vi "BiasPreamp.vi"(0 "VISA resource name":refnum<visa-resource-name>="COM8", 1 "CHANGE SENS?":bool=TRUE, 2 "Sensitivity":T1(ring)=enum."100nA/V", 3 "Bias on":bool=TRUE, 4 "Bias Voltage (mv)":i32=-25) -> ()   [LabVIEW 2013]
uses:
  <vilib>/Instr/_visa.llb/VISA Configure Serial Port (Instr).vi
panel:
  in  "flow control":u16(ring) items=["None"=0, "XON/XOFF"=1, "RTS/CTS"=2, "DTR/DSR"=4]
  in  "stop bits":u16(ring)=10 items=["1.0"=10, "1.5"=15, "2.0"=20]
  in  "parity":u16(ring) items=["None", "Odd", "Even", "Mark", "Space"]
  in  "data bits":u16=8 min=5 max=8 step=1
  in  "baud rate":u32=9600
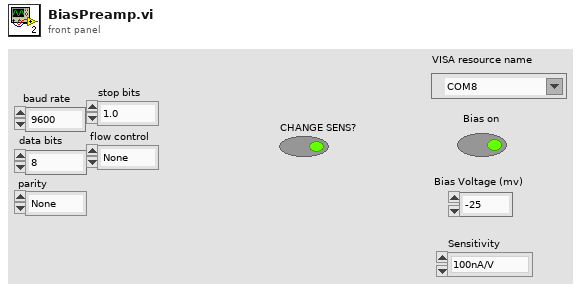
[diagram p1: front panel]
types:
  T1 = enum16{"1pA/V", "2pA/V", "5pA/V", "10pA/V", "20pA/V", "50pA/V", "100pA/V", "200pA/V", "500pA/V", "1nA/V", "2nA/V", "5nA/V", "10nA/V", "20nA/V", "50nA/V", "100nA/V", "200nA/V", "500nA/V", "1uA/V", "2uA/V", "5uA/V", "10uA/V", "20uA/V", "50uA/V", "100uA/V", "200uA/V", "500uA/V", "1mA/V"}
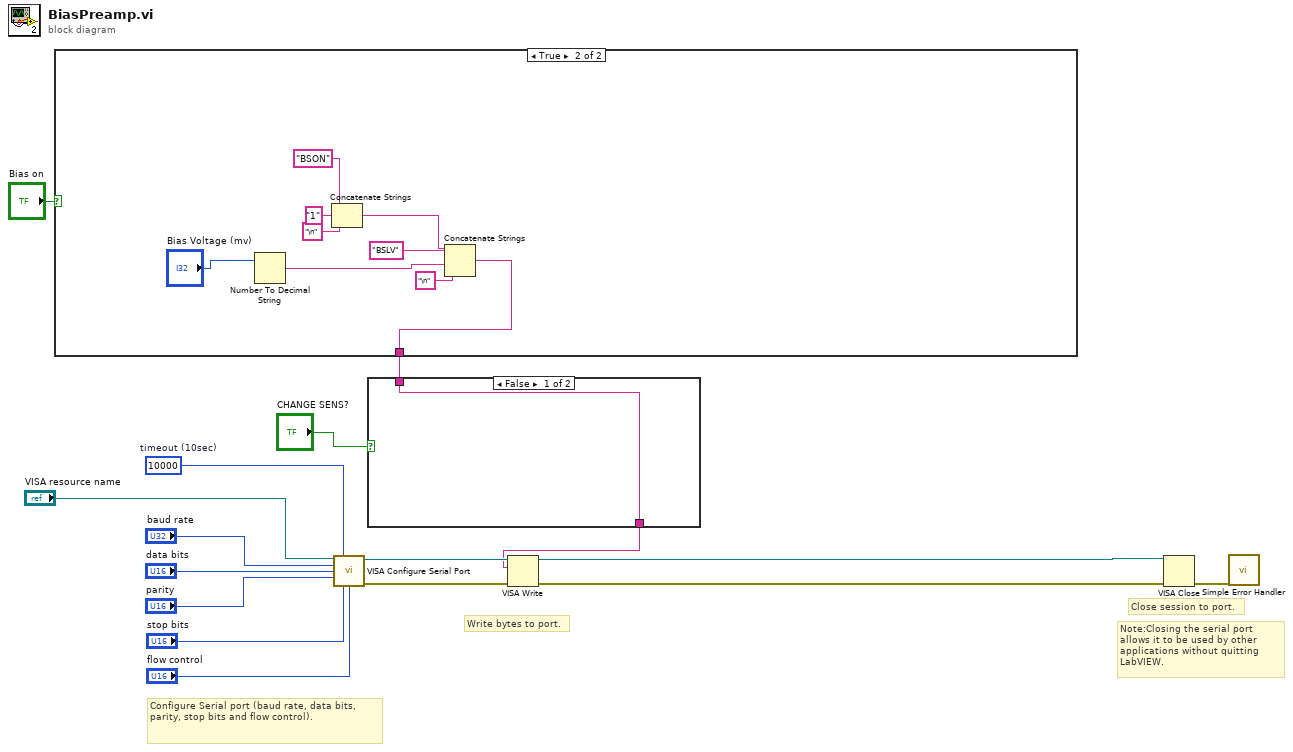
[diagram p0: block diagram]
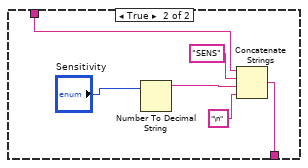
[diagram p2: hidden frame]
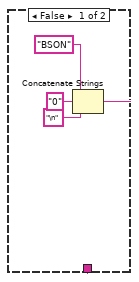
[diagram p3: hidden frame]
diagram:
  w10 = u32 10000  # timeout (10sec)
  # "Write bytes to port."
  # "Note:Closing the serial port allows it to be used by other applications without quitting LabVIEW."
  # "Configure Serial port (baud rate, data bits, parity, stop bits and flow control)."
  # "Close session to port."
  n1 = case shown="True" "Bias on" {
    tunnel: [w17 w22] -> w3
    frame False {
      n2 = Concatenate Strings("BSON", "0" ("string"), "\n" ("string")) -> (w17:string)
    }
    frame True {
      n3 = Number To Decimal String(number="Bias Voltage (mv)") -> (decimal integer string=w23:string)  [unwired: 1 in]
      n4 = Concatenate Strings("BSON", "1" ("string"), "\n" ("string")) -> (w21:string)
      n5 = Concatenate Strings(w21, "BSLV", w23, "\n" ("string")) -> (w22:string)
    }
  }
  n6 = call-poly "VISA Configure Serial Port"("VISA resource name"="VISA resource name", "timeout (10sec)"=w10, "baud rate (9600)"="baud rate", "data bits (8)"="data bits", "parity (0:none)"="parity", "stop bits (10: 1 bit)"="stop bits", "flow control (0:none)"="flow control") -> ("VISA resource name out"=w13:refnum<visa-resource-name>, "error out"=w14:errorcluster)  [unwired: 2 in, 5 out]
  n7 = case shown="False" "CHANGE SENS?" {
    tunnel: w3 -> [w30 w32]
    tunnel: [w30 w31] -> w2
    frame False {
    }
    frame True {
      n8 = Number To Decimal String(number="Sensitivity") -> (decimal integer string=w34:string)  [unwired: 1 in]
      n9 = Concatenate Strings(w32, "SENS" ("string"), w34, "\n" ("string")) -> (w31:string)
    }
  }
  n10 = VISA Write(VISA resource name=w13, write buffer=w2, error in (no error)=w14) -> (VISA resource name out=w6:refnum<visa-resource-name>, error out=w5:errorcluster)  [unwired: 1 out]
  n11 = VISA Close(VISA resource name=w6, error in (no error)=w5) -> (error out=w12:errorcluster)
  n12 = call <vilib>:"Simple Error Handler.vi"("error in (no error)"=w12) -> ()  [unwired: 1 in, 8 out]
